vi "Update Enum Conversions.vi"(6 "Built Enumeration":T1, 7 "App":refnum<vi>, 8 "error in (no error)":errorcluster, 10 "Values":i32[](array[numeric]), 11 "LV-Protoc in":refnum<class "LV-Protoc.lvclass">) -> (0 "error out":errorcluster, 3 "LV-Protoc out":refnum<class "LV-Protoc.lvclass">)   [LabVIEW 2020, in "LV-Protoc.lvlib" / "LV-Protoc.lvclass"]
uses:
  LV-Protoc.lvclass
  Enumeration Paths.ctl
  <vilib>/Utility/traverseref.llb/TRef TravTarget.ctl
  LV-Protoc.lvlib
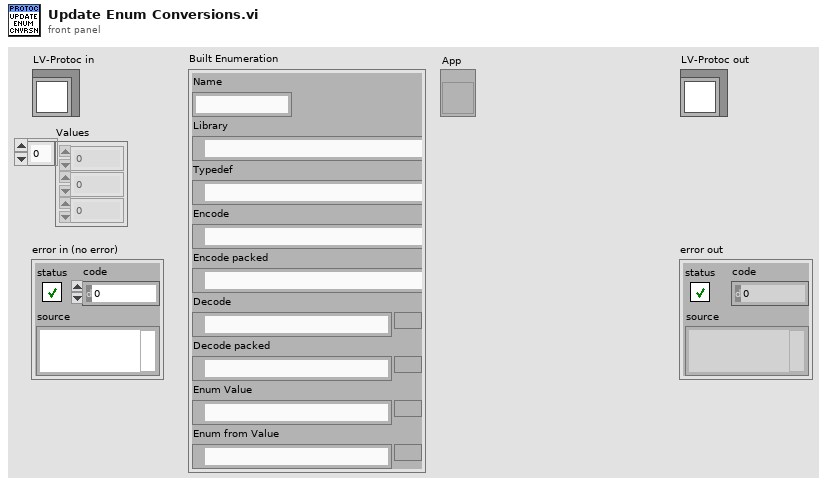
[diagram p1: front panel]
types:
  T1 = typedef "LV-Protoc.lvlib/Enumeration Paths.ctl" = cluster{"Name":string, "Library":path, "Typedef":path, "Encode":path, "Encode packed":path, "Decode":path, "Decode packed":path, "Enum Value":path, "Enum from Value":path}
  T2 = typedef "TRef TravTarget.ctl" = enum16{"FP", "BD", "Other"}
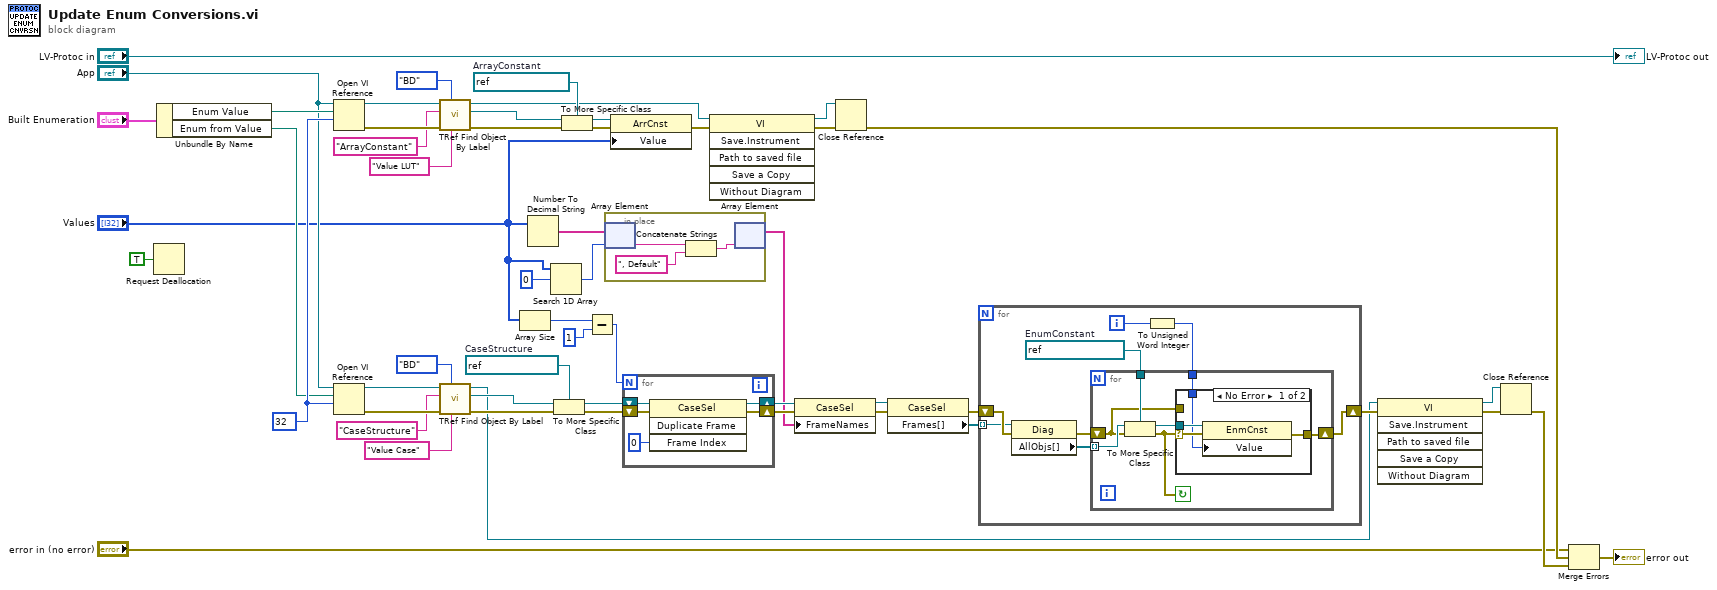
[diagram p0: block diagram]
diagram:
  w41 = refnum<vi> refnum  # ArrayConstant
  w31 = refnum<vi> refnum  # CaseStructure
  w51 = 32 ("options")
  n1 = Request Deallocation(TRUE ("flag")) -> ()
  n2 = Unbundle By Name("Built Enumeration") -> ("Enum Value"=w7:path, "Enum from Value"=w6:path)
  n3 = Open VI Reference(application reference (local)="App", vi path=w7, options=w51) -> (vi reference=w50:refnum<vi>, error out=w52:errorcluster)  [unwired: 3 in]
  n4 = Open VI Reference(application reference (local)="App", vi path=w6, options=w51) -> (vi reference=w43:refnum<vi>, error out=w53:errorcluster)  [unwired: 3 in]
  n5 = call <vilib>:"TRef Find Object By Label.vi"("Label"="Value LUT", "Traverse Target"=TRef_TravTarget."BD", "error in (no error)"=w52, "Class Name"="ArrayConstant", "VI Ref"=w50) -> ("error out"=w40:errorcluster, "Found Obj Ref"=w42:refnum<vi>, "dup VI Ref"=w36:refnum<vi>)  [unwired: 3 in, 1 out]
  n6 = call <vilib>:"TRef Find Object By Label.vi"("Label"="Value Case", "Traverse Target"=TRef_TravTarget."BD", "error in (no error)"=w53, "Class Name"="CaseStructure", "VI Ref"=w43) -> ("error out"=w33:errorcluster, "Found Obj Ref"=w32:refnum<vi>, "dup VI Ref"=w13:refnum<vi>)  [unwired: 3 in, 1 out]
  n7 = Array Size(array="Values") -> (size(s)=w30:i32)
  n8 = Number To Decimal String(number="Values") -> (decimal integer string=w24:string[])  [unwired: 1 in]
  n9 = Search 1D Array(1D array="Values", element=0) -> (index of element=w1:i32)  [unwired: 1 in]
  n10 = To More Specific Class(target class=w31, reference=w32, error in=w33) -> (specific class reference=w21:refnum<vi>, error out=w22:errorcluster)
  n11 = To More Specific Class(target class=w41, reference=w42, error in=w40) -> (specific class reference=w39:refnum<vi>, error out=w38:errorcluster)
  n12 = Subtract(x=w30, y=1) -> (x-y=w28:i32)
  n13 = in-place {
    n14 = in-place-array #1(w24, w1) -> (w56:string)
    n15 = Concatenate Strings(w56, ", Default" ("string")) -> (w54:string)
    n16 = in-place-array #1(w54) -> (w23:string[])  [unwired: 1 out]
  }
  n17 = property class="ArrCnst"(reference=w39, error in=w38, "Value"="Values") -> (error out=w37:errorcluster)  [unwired: 1 out]
  n18 = for {
    N: w28 -> [_]
    shift-right: [w58] -> w27
    shift-left: w21 -> [w60]
    shift-right: [w57] -> w26
    shift-left: w22 -> [w61]
    n19 = invoke class="CaseSel" method="Duplicate Frame"(reference=w60, error in=w61, "Frame Index"=u32 0) -> (reference out=w58:refnum<vi>, error out=w57:errorcluster)  [unwired: 1 in, 2 out]
  }
  n20 = invoke class="VI" method="Save.Instrument"(reference=w36, error in=w37) -> (reference out=w34:refnum<vi>, error out=w35:errorcluster)  [unwired: 4 in, 4 out]
  n21 = property class="CaseSel"(reference=w27, error in=w26, "FrameNames"=w23) -> (reference out=w20:refnum<vi>, error out=w19:errorcluster)
  n22 = Close Reference(reference=w34, error in (no error)=w35) -> (error out=w12:errorcluster)
  n23 = property class="CaseSel"(reference=w20, error in=w19) -> (error out=w18:errorcluster, "Frames[]"=w17:refnum<vi>[])  [unwired: 1 out]
  n24 = for {
    shift-right: [w64] -> w16
    shift-left: w18 -> [w69]
    tunnel: w17 -> [w68] mode=indexing
    i -> [w62]
    w65 = refnum<vi> refnum  # EnumConstant
    n25 = property class="Diag"(reference=w68, error in=w69) -> (error out=w66:errorcluster, "AllObjs[]"=w67:refnum<vi>[])  [unwired: 1 out]
    n26 = To Unsigned Word Integer(number=w62) -> (unsigned 16bit integer=w63:u16)
    n27 = for {
      tunnel: w67 -> [w76] mode=indexing
      shift-right: [w71] -> w64
      shift-left: w66 -> [w70]
      tunnel: w65 -> [w75]
      tunnel: w63 -> [w72]
      stop <- w73 continue-if-true
      n28 = To More Specific Class(target class=w75, reference=w76, error in=w70) -> (specific class reference=w74:refnum<vi>, error out=w73:errorcluster)
      n29 = case shown="No Error" w73 {
        selector: w73 -> [w79 _]
        tunnel: w74 -> [w80 _]
        tunnel: w72 -> [w78 _]
        tunnel: [w77 w81] -> w71
        tunnel: w70 -> [_ w81]
        frame No Error {
          n30 = property class="EnmCnst"(reference=w80, error in=w79, "Value"=w78) -> (error out=w77:errorcluster)  [unwired: 1 out]
        }
        frame Error {
        }
      }
    }
  }
  n31 = invoke class="VI" method="Save.Instrument"(reference=w13, error in=w16) -> (reference out=w14:refnum<vi>, error out=w15:errorcluster)  [unwired: 4 in, 4 out]
  n32 = Close Reference(reference=w14, error in (no error)=w15) -> (error out=w11:errorcluster)
  n33 = Merge Errors("error in (no error)", w12, w11) -> (→"error out":errorcluster)
  "LV-Protoc out" <- "LV-Protoc in"
